vi "Add Minor Frame.vi"(7 "frameTime uS (200)":i32=200, 8 "error in":errorcluster, 9 "Scheduled Message Config in":T1[](array[typedef]), 10 "name":string, 11 "BusController in":refnum<k24>) -> (0 "error out":errorcluster, 2 "new Minor Frame":refnum<k24>, 3 "BusController out":refnum<k24>)   [LabVIEW 2020, in "Ballard_1553_Hardware_ni.lvlib"]
uses:
  Ballard_1553_Hardware_ni.lvlib
  C:/Users/Administrator/Desktop/GIT/Ballard-MIL-STD-1553-Custom-Device/Source/System Explorer/SubVIs/Parse XML Ballard/1.2/BTIXML_SerDes.dll
  Ballard-MIL-STD-1553-Custom-Device/Source/System Explorer/SubVIs/Parse XML Ballard/1.2/BTIXML_SerDes.dll
  _typedefs/schedItem1553_type.ctl
  _typedefs/frame_entry_type.ctl
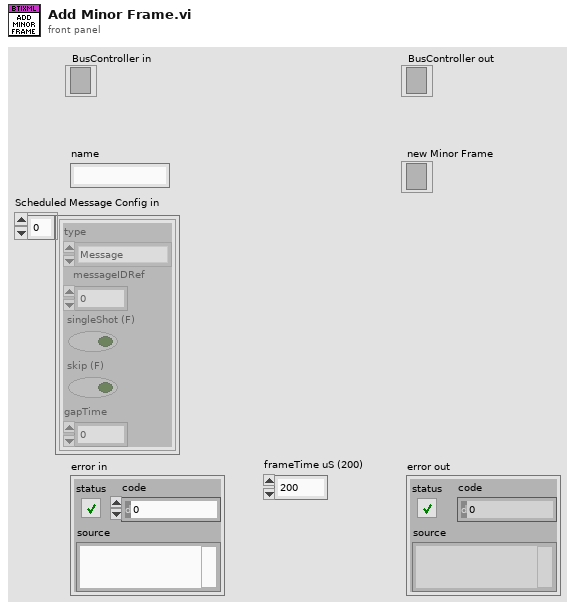
[diagram p1: front panel]
types:
  T1 = typedef "Ballard_1553_Hardware_ni.lvlib/schedItem1553_type.ctl" = cluster{"type":T2, "messageIDRef":i32, "singleShot (F)":bool, "skip (F)":bool, "gapTime":dbl}
  T2 = typedef "Ballard_1553_Hardware_ni.lvlib/frame_entry_type.ctl" = enum16{"Message", "Gap", "Pulse", "Log", "Pause", "Restart", "Halt"}
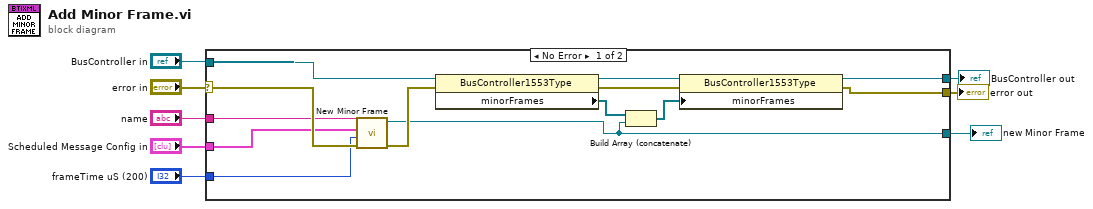
[diagram p0: block diagram]
diagram:
  n1 = case shown="No Error" "error in" {
    selector: "error in" -> [w14 w22]
    tunnel: [w18 w22] -> w8
    tunnel: [w19 w23] -> w7
    tunnel: "BusController in" -> [w21 w23]
    tunnel: [w12 _] -> w4
    tunnel: "name" -> [w11 _]
    tunnel: "Scheduled Message Config in" -> [w10 _]
    tunnel: "frameTime uS (200)" -> [w9 _]
    frame No Error {
      n2 = call "New Minor Frame.vi"("error in"=w14, "frameTime uS (200)"=w9, "Scheduled Message Config in"=w10, "name"=w11) -> ("error out"=w13:errorcluster, "new minor frame"=w12:refnum<k24>)  [unwired: 6 in]
      n3 = property class="BusController1553Type"(reference=w21, error in=w13) -> (reference out=w20:refnum<k24>, error out=w17:errorcluster, "minorFrames"=w16:refnum<k24>[])
      n4 = Build Array (concatenate)(w16, w12) -> (w15:refnum<k24>[])
      n5 = property class="BusController1553Type"(reference=w20, error in=w17, "minorFrames"=w15) -> (reference out=w19:refnum<k24>, error out=w18:errorcluster)
    }
    frame Error {
    }
  }
  "error out" <- w8
  "BusController out" <- w7
  "new Minor Frame" <- w4
